vi "Command Type.vi"(11 "Command Config in":refnum<class "Command Config.lvclass">) -> (2 "Command Type":string)   [LabVIEW 2020, in "VolatusSeqConfig.lvlib" / "Command Config.lvclass"]
uses:
  Command Config.lvclass
  Command Config.lvclass/Command Config.ctl
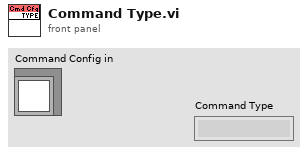
[diagram p1: front panel]
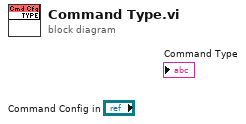
[diagram p0: block diagram]
diagram:
